vi "Wizard Global Variable.vi"() -> ()   [LabVIEW 2014]
panel:
  in  "no. Imported Var":i32
  in  "Second Decision":enum32{"Database Ready", "Make Database"}(ring)
  out "Finish?":bool
  out "Binding?":bool
  in  "First Decision":enum32{"Create", "Manage"}(ring)
  out "SV Created":bool
  out "SV Path":path
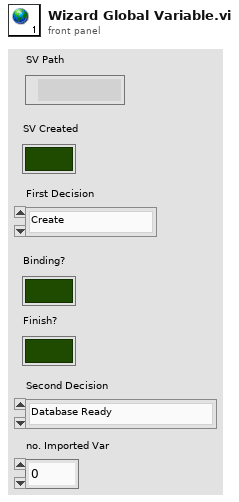
[diagram p1: front panel]
diagram:
